vi "Set Port Config.vi"(8 "error in (no error)":errorcluster, 10 "Port Config":T1={"Baud (115200)"=115200, "Data Bits (8)"=8, "Stop Bits (1)"=10, "Flow Control"=0, "LineTerm (\\n)"="\n", "Timeout ms (10000)"=10000, "Parity (None)"=enum."None"} {"Flow Control" items=["None", "XON/XOFF", "RTS/CTS", "XON/XOFF & RTS/CTS", "DTR/DSR", "XON/XOFF & DTR/DSR"]; "Stop Bits (1)" items=["1.0"=10, "1.5"=15, "2.0"=20]}, 11 "Serial Client in":refnum<class "Serial Client.lvclass">) -> (0 "error out":errorcluster, 3 "Serial Client out":refnum<class "Serial Client.lvclass">)   [LabVIEW 2020, in "Stream-Serial.lvlib" / "Serial Client.lvclass"]
doc: "Sets the serial port parameters to be used when opening the port. The <b>LineTerm</b> parameter only applies when the Connection is set to LineTerm Mode when initialized.\n\nTrying to set the Port Config while the connection is open will return an error and ignore the change. Be sure to <b>Close</b> an open connection before updating port configuration."
uses:
  Serial Client.lvclass
  Serial Client.lvclass/Serial Client.ctl
  <vilib>/IlluminatedG/lv-stream/Connection/Connection.lvclass
  C:/Program Files (x86)/National Instruments/LabVIEW 2020/vi.lib/IlluminatedG/lv-stream/Connection/Connection.lvclass
  C:/Program Files (x86)/National Instruments/LabVIEW 2020/vi.lib/IlluminatedG/lv-stream/Endpoint/Endpoint.lvclass
  C:/dev/IlluminatedG/lv-stream-serial/Stream-Serial/Serial Client/Serial Client.lvclass
  Flow Control.ctl
  Port Config.ctl
  Stop Bits.ctl
  Parity.ctl
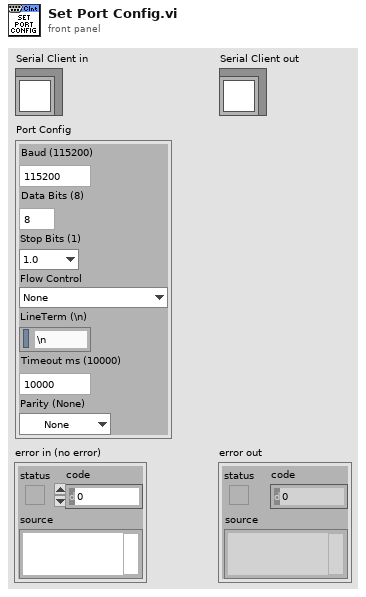
[diagram p1: front panel]
types:
  T1 = typedef "Stream-Serial.lvlib/Serial Client.lvclass/Port Config.ctl" = cluster{"Baud (115200)":u32, "Data Bits (8)":u8, "Stop Bits (1)":T2, "Flow Control":T3, "LineTerm (\\n)":string, "Timeout ms (10000)":i32, "Parity (None)":T4}
  T2 = typedef "Stream-Serial.lvlib/Serial Client.lvclass/Stop Bits.ctl" = u16
  T3 = typedef "Stream-Serial.lvlib/Serial Client.lvclass/Flow Control.ctl" = u16
  T4 = typedef "Stream-Serial.lvlib/Serial Client.lvclass/Parity.ctl" = enum16{"None", "Odd", "Even", "Mark", "Space"}
  T5 = typedef "Stream.lvlib/Connection.lvclass/State.ctl" = enum16{"Closed", "Idle", "Connecting", "Connected", "Shutdown"}
  T6 = typedef "Stream-Serial.lvlib/Serial Client.lvclass/Ref Data.ctl" = cluster{"Stream":refnum<class "Serial Stream.lvclass">, "Client Loop":refnum<vi>, "Port Config":T1, "VISA Resource":refnum<visa-resource-name>}
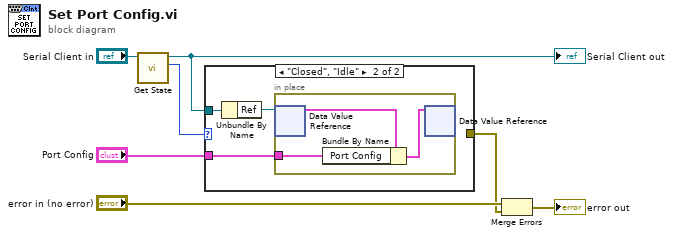
[diagram p0: block diagram]
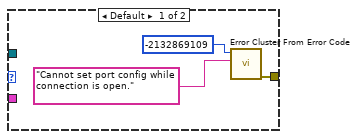
[diagram p2: hidden frame]
diagram:
  n1 = call <vilib>:"Get State.vi"("Connection in"="Serial Client in") -> ("State"=w1:T5, "Connection out"=w2:refnum<class "Serial Client.lvclass">)  [unwired: 8 in, 1 out]
  "Serial Client out" <- w2
  n2 = case shown="\"Closed\", \"Idle\"" w1 {
    tunnel: "Port Config" -> [_ w12]
    tunnel: w2 -> [_ w11]
    tunnel: [w9 _] -> w4
    frame Default {
      n3 = call <vilib>:"Error Cluster From Error Code.vi"("error message (\"\")"="Cannot set port config while connection is open.", "error code (0)"=-2132869109) -> ("error out"=w9:errorcluster)  [unwired: 7 in]
    }
    frame "Closed", "Idle" {
      n4 = Unbundle By Name(w11) -> ("Ref"=w13:refnum<data-value>)
      n5 = in-place {
        in-place-border: w12 -> [w14]
        n6 = in-place-dvr #1(w13) -> (w16:T6)  [unwired: 1 out]
        n7 = Bundle By Name(cluster=w16, "Port Config"=w14) -> (w15:T6)
        n8 = in-place-dvr #1(w15) -> ()  [unwired: 2 out]
      }
    }
  }
  n9 = Merge Errors("error in (no error)", w4) -> (→"error out":errorcluster)
